vi "Actor Teardown.vi"(10 "Error":errorcluster, 11 "Dev Actor in":refnum<class "Dev Actor.lvclass">) -> (0 "error out":errorcluster, 2 "Teardown?":bool)   [LabVIEW 2021, in "Dev Actor.lvlib" / "Dev Actor.lvclass"]
uses:
  Dev Actor.lvclass
  Dev Actor.lvclass/Dev Actor.ctl
  LVCAM/LVCAM/Actor/Actor.lvclass
  Panel/Panel.lvclass
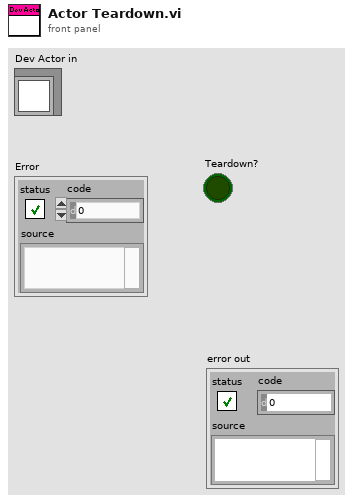
[diagram p1: front panel]
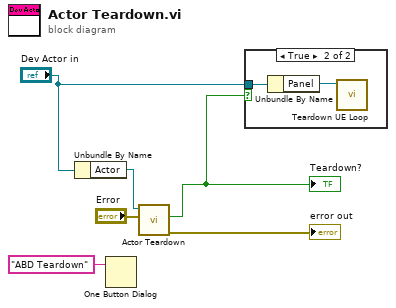
[diagram p0: block diagram]
diagram:
  n1 = Unbundle By Name("Dev Actor in") -> ("Actor"=w3:refnum<class "Actor.lvclass">)
  n2 = One Button Dialog(message="ABD Teardown") -> ()  [unwired: 1 in, 1 out]
  n3 = call-dynamic "Actor Teardown.vi"("Error"="Error", "Actor in"=w3) -> ("error out"=→"error out":errorcluster, "Teardown?"=w2:bool)  [unwired: 8 in]
  "Teardown?" <- w2
  n4 = case shown="True" w2 {
    tunnel: "Dev Actor in" -> [_ w8]
    frame False {
    }
    frame True {
      n5 = Unbundle By Name(w8) -> ("Panel"=w7:refnum<class "Panel.lvclass">)
      n6 = call-dynamic "Teardown UE Loop.vi"("Panel in"=w7) -> ()  [unwired: 10 in, 1 out]
    }
  }
